vi "Recursive_GetDiagrams[].vi"(8 "error in (no error)":errorcluster, 11 "AllObjs[]":refnum<vi>[](array[refnum])) -> (0 "error out":errorcluster, 3 "Diagrams":refnum<vi>[](array[refnum]))   [LabVIEW 2014]
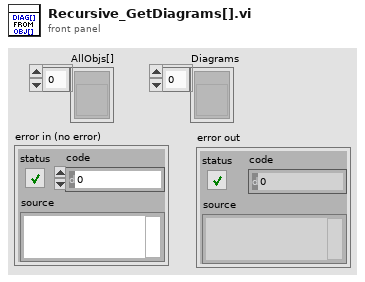
[diagram p1: front panel]
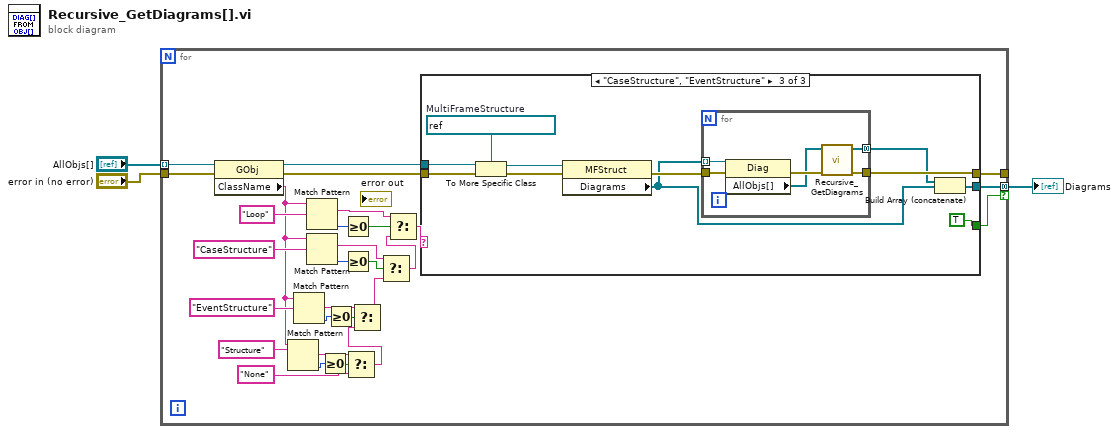
[diagram p0: block diagram]
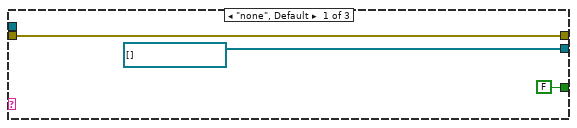
[diagram p2: hidden frame]
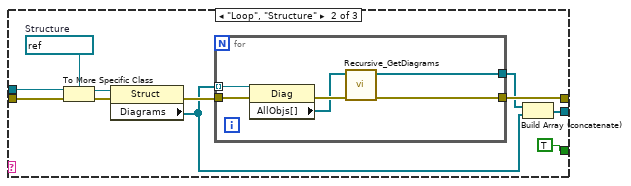
[diagram p3: hidden frame]
diagram:
  n1 = for {
    tunnel: [w28] -> w3 mode=concatenating if=w13
    tunnel: "AllObjs[]" -> [w27] mode=indexing
    tunnel: "error in (no error)" -> [w25]
    tunnel: [w24] -> _
    n2 = property class="GObj"(reference=w27, error in=w25) -> (reference out=w26:refnum<vi>, error out=w29:errorcluster, "ClassName"=w4:string)
    n3 = Match Pattern(string=w4, regular expression="Structure" ("search string")) -> (match substring=w23:string, offset past match=w22:i32)  [unwired: 1 in, 2 out]
    n4 = Match Pattern(string=w4, regular expression="EventStructure" ("search string")) -> (match substring=w8:string, offset past match=w9:i32)  [unwired: 1 in, 2 out]
    n5 = Match Pattern(string=w4, regular expression="Loop" ("search string")) -> (match substring=w15:string, offset past match=w31:i32)  [unwired: 1 in, 2 out]
    n6 = Match Pattern(string=w4, regular expression="CaseStructure" ("search string")) -> (match substring=w17:string, offset past match=w32:i32)  [unwired: 1 in, 2 out]
    n7 = Greater Or Equal To 0?(x=w22) -> (x >= 0?=w21:bool)
    n8 = Greater Or Equal To 0?(x=w9) -> (x >= 0?=w10:bool)
    n9 = Greater Or Equal To 0?(x=w31) -> (x >= 0?=w16:bool)
    n10 = Greater Or Equal To 0?(x=w32) -> (x >= 0?=w19:bool)
    n11 = Select(t=w23, s=w21, f="None" ("search string")) -> (s? t:f=w7:string)
    n12 = Select(t=w8, s=w10, f=w7) -> (s? t:f=w6:string)
    n13 = Select(t=w17, s=w19, f=w6) -> (s? t:f=w18:string)
    n14 = Select(t=w15, s=w16, f=w18) -> (s? t:f=w14:string)
    n15 = case shown="\"CaseStructure\", \"EventStructure\"" w14 {
      tunnel: w29 -> [w34 w43 w61]
      tunnel: [refnum<vi>[] [] ("Diagrams") w39 w57] -> w28
      tunnel: w26 -> [_ w42 w60]
      tunnel: [w34 w40 w58] -> w24
      tunnel: [FALSE TRUE TRUE] -> w13
      frame "none", Default {
      }
      frame "Loop", "Structure" {
        w46 = refnum<vi> refnum  # Structure
        n16 = To More Specific Class(target class=w46, reference=w42, error in=w43) -> (specific class reference=w45:refnum<vi>, error out=w44:errorcluster)
        n17 = property class="Struct"(reference=w45, error in=w44) -> (error out=w41:errorcluster, "Diagrams"=w37:refnum<vi>[])  [unwired: 1 out]
        n18 = for {
          tunnel: [w50] -> w38
          tunnel: w37 -> [w48] mode=indexing
          tunnel: w41 -> [w52]
          tunnel: [w51] -> w40
          n19 = property class="Diag"(reference=w48, error in=w52) -> (error out=w49:errorcluster, "AllObjs[]"=w47:refnum<vi>[])  [unwired: 1 out]
          n20 = call "Recursive_GetDiagrams.vi"("error in (no error)"=w49, "AllObjs[]"=w47) -> ("error out"=w51:errorcluster, "Diagrams"=w50:refnum<vi>[])  [unwired: 8 in]
        }
        n21 = Build Array (concatenate)(w38, w37) -> (w39:refnum<vi>[])
      }
      frame "CaseStructure", "EventStructure" {
        w53 = refnum<vi> refnum  # MultiFrameStructure
        n22 = To More Specific Class(target class=w53, reference=w60, error in=w61) -> (specific class reference=w63:refnum<vi>, error out=w62:errorcluster)
        n23 = property class="MFStruct"(reference=w63, error in=w62) -> (error out=w59:errorcluster, "Diagrams"=w55:refnum<vi>[])  [unwired: 1 out]
        n24 = for {
          tunnel: [w67] -> w56 mode=concatenating
          tunnel: w55 -> [w65] mode=indexing
          tunnel: w59 -> [w69]
          tunnel: [w68] -> w58
          n25 = property class="Diag"(reference=w65, error in=w69) -> (error out=w66:errorcluster, "AllObjs[]"=w64:refnum<vi>[])  [unwired: 1 out]
          n26 = call "Recursive_GetDiagrams.vi"("error in (no error)"=w66, "AllObjs[]"=w64) -> ("error out"=w68:errorcluster, "Diagrams"=w67:refnum<vi>[])  [unwired: 8 in]
        }
        n27 = Build Array (concatenate)(w56, w55) -> (w57:refnum<vi>[])
      }
    }
  }
  "Diagrams" <- w3
